vi "createLabVIEWTypedefs.vi"(8 "error in (no error)":errorcluster, 10 "targetBasePath":path, 11 "IDLFile in":refnum<class "IDLFile.lvclass">) -> (0 "error out":errorcluster, 3 "IDLFile out":refnum<class "IDLFile.lvclass">)   [LabVIEW 2016, in "IDLFile.lvclass"]
uses:
  IDLFile.lvclass
  IDLFile.lvclass/IDLFile.ctl
  Module/Module.lvclass
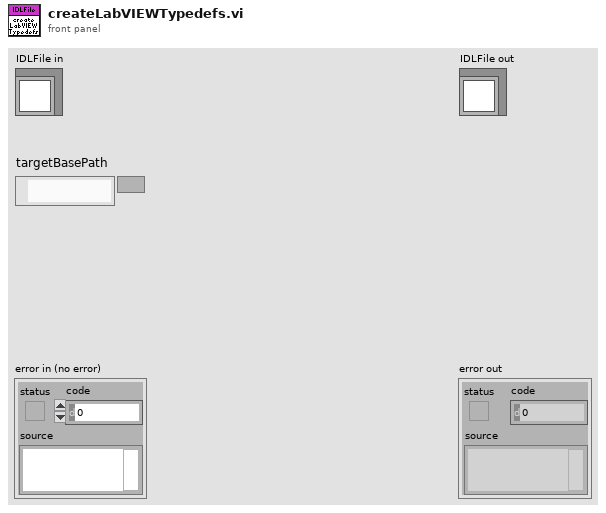
[diagram p1: front panel]
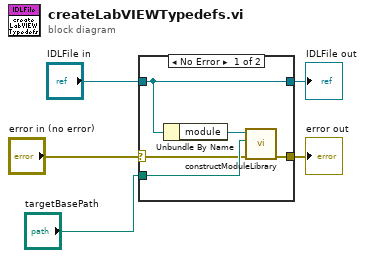
[diagram p0: block diagram]
diagram:
  n1 = case shown="No Error" "error in (no error)" {
    selector: "error in (no error)" -> [w7 w12]
    tunnel: [w6 w12] -> w4
    tunnel: [w10 w11] -> w2
    tunnel: "IDLFile in" -> [w10 w11]
    tunnel: "targetBasePath" -> [w8 _]
    frame No Error {
      n2 = Unbundle By Name(w10) -> ("module"=w9:refnum<class "Module.lvclass">)
      n3 = call "constructModuleLibrary.vi"("error in (no error)"=w7, "targetBasePath"=w8, "Module in"=w9) -> ("error out"=w6:errorcluster)  [unwired: 7 in, 1 out]
    }
    frame Error {
    }
  }
  "error out" <- w4
  "IDLFile out" <- w2
